vi "ROS_Subscribers.vi"() -> ()   [LabVIEW 2016]
doc: "The ROS Subscriber subscribes to two topics, the unicorn current state and the intention variable from the local planner."
uses:
  builds/UnicornMain/UnicornRIO1/ROS for LabVIEW/home/lvuser/natinst/bin/user.lib/ROS for LabVIEW Software/ROS/Code/Console/Servers/ServerSubs/TopicDef.ctl
  builds/UnicornMain/UnicornRIO1/ROS for LabVIEW/home/lvuser/natinst/bin/user.lib/ROS for LabVIEW Software/ROS/Code/SubVIs/_ROSDirection.ctl
  builds/ROS_Test1/UnicornRIO1/ROS for LabVIEW/home/lvuser/natinst/bin/user.lib/ROS for LabVIEW Software/ROS/Code/_ROSDefinition.vi
  GlobalVI.vi
  documentation/ROS for LabVIEW Software/ROS/MessageParsing/std_msgs/subs/parse_u32_scalar.vi
  builds/UnicornMain/UnicornRIO1/ROS for LabVIEW/home/lvuser/natinst/bin/user.lib/ROS for LabVIEW Software/ROS/MessageParsing/std_msgs/subs/parse_i32_scalar.vi
panel:
  out "PickingRoutine":u32
  out "\\TX2_unicorn_state":i32
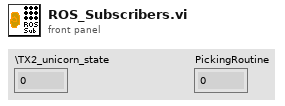
[diagram p1: front panel]
types:
  T1 = typedef "TopicDef.ctl" = cluster{"Topic":string, "Type":string, "Action":T2, "Update (ms)":u16, "queue size":u16}
  T2 = typedef "_ROSDirection.ctl" = enum16{"Node", "Publisher", "Subscriber", "ServiceClient", "ServiceProvider"}
  T3 = typedef "_ROSControl.ctl" = cluster{"topic port":u16, "Node":string, "topic":string, "type":string, "node port":u16, "error ":errorcluster, "Direction":T2, "Update (ms)":u16, "FIFO size":u16}
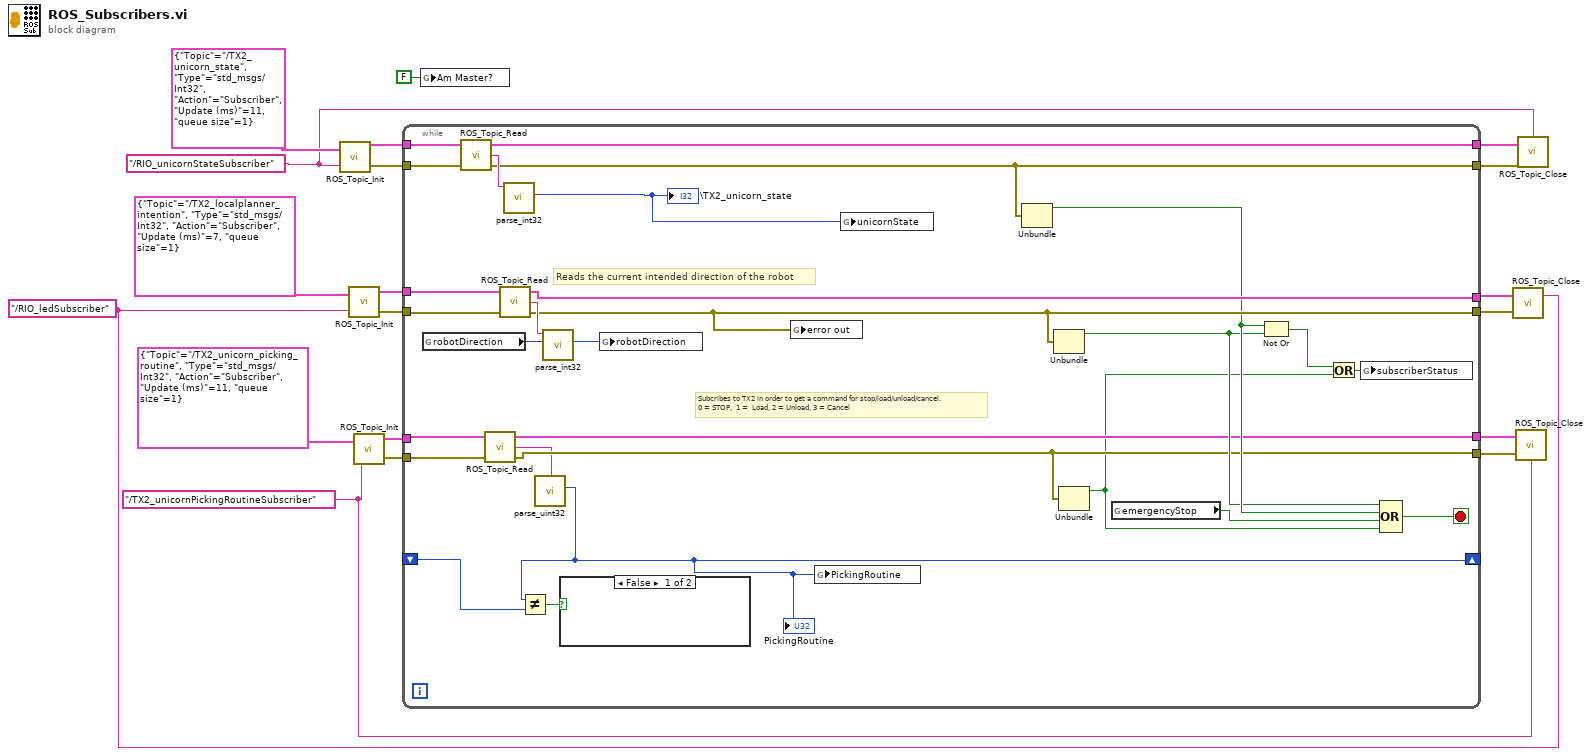
[diagram p0: block diagram]
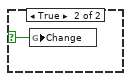
[diagram p2: hidden frame]
diagram:
  w1 = "/TX2_unicornPickingRoutineSubscriber" ("node")
  w13 = "/RIO_ledSubscriber" ("node")
  w15 = "/RIO_unicornStateSubscriber" ("node")
  n1 = call "ROS_Topic_Init.vi"("Definitions"=T1 {"Topic"="/TX2_unicorn_state", "Type"="std_msgs/Int32", "Action"=enum."Subscriber", "Update (ms)"=11, "queue size"=1}, "node"=w15) -> ("ROS out"=w18:T3, "error out"=w7:errorcluster)  [unwired: 1 in]
  n2 = call "ROS_Topic_Init.vi"("Definitions"=T1 {"Topic"="/TX2_localplanner_intention", "Type"="std_msgs/Int32", "Action"=enum."Subscriber", "Update (ms)"=7, "queue size"=1}, "node"=w13) -> ("ROS out"=w12:T3, "error out"=w8:errorcluster)  [unwired: 1 in]
  n3 = call "ROS_Topic_Init.vi"("Definitions"=T1 {"Topic"="/TX2_unicorn_picking_routine", "Type"="std_msgs/Int32", "Action"=enum."Subscriber", "Update (ms)"=11, "queue size"=1}, "node"=w1) -> ("ROS out"=w5:T3, "error out"=w4:errorcluster)  [unwired: 1 in]
  n4 = while {
    tunnel: w18 -> [w47]
    tunnel: [w45] -> w16
    tunnel: w7 -> [w46]
    tunnel: [w37] -> w17
    tunnel: w12 -> [w42]
    tunnel: w8 -> [w41]
    tunnel: [w36] -> w11
    tunnel: [w40] -> w10
    tunnel: w5 -> [w31]
    tunnel: w4 -> [w30]
    tunnel: [w29] -> w3
    tunnel: [w28] -> w2
    shift-right: [w20] -> _
    shift-left: _ -> [w23]
    stop <- w35 stop-if-true
    # "Subcribes to TX2 in order to get a command for stop/load/unload/cancel. \n0 = STOP,  1 =  Load, 2 = Unload, 3 = Cancel"
    # "Reads the current intended direction of the robot"
    n5 = global read "GlobalVI.vi" "robotDirection"() -> (w38:i32)
    n6 = call "ROS_Topic_Read.vi"("error in (no error)"=w46, "ROS in"=w47) -> ("error out"=w37:errorcluster, "Reply"=w44:string, "ROS out"=w45:T3)  [unwired: 1 in]
    n7 = call "ROS_Topic_Read.vi"("error in (no error)"=w30, "ROS in"=w31) -> ("error out"=w28:errorcluster, "Reply"=w24:string, "ROS out"=w29:T3)  [unwired: 1 in]
    n8 = call "ROS_Topic_Read.vi"("error in (no error)"=w41, "ROS in"=w42) -> ("error out"=w36:errorcluster, "Reply"=w43:string, "ROS out"=w40:T3)  [unwired: 1 in]
    n9 = call-poly "parse_int32.vi"("msg in"=w44) -> ("number"=w22:i32)  [unwired: 4 in, 2 out]
    "\\TX2_unicorn_state" <- w22
    n10 = call-poly <userlib>:"parse_uint32.vi"("msg in"=w24) -> ("number"=w20:u32)  [unwired: 4 in, 2 out]
    "PickingRoutine" <- w20
    n11 = Not Equal?(x=w20, y=w23) -> (x != y?=w21:bool)
    n12 = call-poly "parse_int32.vi"("type"=w38, "msg in"=w43) -> ("number"=w39:i32)  [unwired: 3 in, 2 out]
    n13 = case shown="False" w21 {
      selector: w21 -> [_ w48]
      frame False {
      }
      frame True {
        n14 = global write "GlobalVI.vi" "Change"(w48) -> ()
      }
    }
    n15 = global write "GlobalVI.vi" "robotDirection"(w39) -> ()
    n16 = global write "GlobalVI.vi" "error out"(w36) -> ()
    n17 = global write "GlobalVI.vi" "PickingRoutine"(w20) -> ()
    n18 = global write "GlobalVI.vi" "unicornState"(w22) -> ()
    n19 = Unbundle(w37) -> ("status"=w33:bool)  [unwired: 2 out]
    n20 = Unbundle(w36) -> ("status"=w32:bool)  [unwired: 2 out]
    n21 = Unbundle(w28) -> ("status"=w25:bool)  [unwired: 2 out]
    n22 = global read "GlobalVI.vi" "emergencyStop"() -> (w34:bool)
    n23 = Not Or(1:w32, 2:w33) -> (0:w26:bool)
    n24 = Or(x=w26, y=w25) -> (x .or. y?=w27:bool)
    n25 = global write "GlobalVI.vi" "subscriberStatus"(w27) -> ()
    n26 = Compound Arithmetic op=OR(w32, w33, w34, w25) -> (w35:bool)
  }
  n27 = global write "_ROSDefinition.vi" "Am Master?"(FALSE ("Am Master?")) -> ()
  n28 = call "ROS_Topic_Close.vi"("error in"=w11, "ROS in"=w10, "node"=w13) -> ()  [unwired: 1 in, 1 out]
  n29 = call "ROS_Topic_Close.vi"("error in"=w2, "ROS in"=w3, "node"=w1) -> ()  [unwired: 1 in, 1 out]
  n30 = call "ROS_Topic_Close.vi"("error in"=w17, "ROS in"=w16, "node"=w15) -> ()  [unwired: 1 in, 1 out]
